vi "AR Drone - Simple Video + Simple nav.vi"() -> ()   [LabVIEW 2014]
doc: "Very simple example showing how to use the base VIs to control the AR Drone and receive and display video data."
uses:
  Others (.ctl)/Control cluster.ctl
  <vilib>/LVH/AR Drone Toolkit/Decode NavData/Typedefs/NavData Demo.ctl
  Global.vi
  <vilib>/LVH/AR Drone Toolkit/AR Drone.lvlib
panel:
  out "error":bool
  out "Take off/Land":bool
  in  "video refresh (ms)":u32=40
  out "Refesh Rate Video Loop (ms) 2":u32
  out "Refesh Rate (ms)":u32=5
  out "Hover":bool
  in  "Tab Control":enum32{"Page 1", "Page 2"}(tab)
  out "B&W":T1(plugin-control)
  out "Raw":picture
  in  "Manual":bool=TRUE
  in  "Setup Parameters":T2={"Drone IP address"="192.168.1.1", "Home IP address"="192.168.1.2", "Flight Mode"=enum."INDOOR MODE", "Mounted Hull"=enum."INDOOR HULL", "Video Camera"=0, "Max Altitude (m)"=3.0, "Max Pitch and Roll Angle (deg)"=8.0, "Max Vertical Speed (m/s)"=0.7, "Max Yaw Speed (deg/s)"=100.0} {"Video Camera" items=["Bottom Camera"=1, "Front Camera"=0, "Front in Bottom"=3, "Bottom in Front"=2]}
  in  "stop":bool
  in  "milliseconds to wait":u32=10
  out "ctr+nav":errorcluster
  out "ctr+nav":i32=2242
  out "Battery Remaining 2":dbl(slide)=55.0 scale=0.0..100.0
  out "NavData Out 2":T3={"control state"=enum."TRANS_LANDING", "battery percentage"=55, "pitch (deg)"=-0.02, "roll (deg)"=0.087, "yaw (deg)"=91.646, "altitude (cm)"=0, "vx (cm/s)?"=0.0, "vy (cm/s)?"=0.0, "vz (cm/s)?"=0.0, "detection cam type"=3}
  out "Control Cluster":T4={"Roll"=0.0, "Pitch"=-0.10223389, "Vertical Speed"=0.0, "Yaw Speed"=0.0} {"Yaw Speed" scale=-1.0..1.0; "Vertical Speed" scale=-1.0..1.0; "Pitch" scale=-1.0..1.0; "Roll" scale=-1.0..1.0}
  in  "Emergency Landing":bool
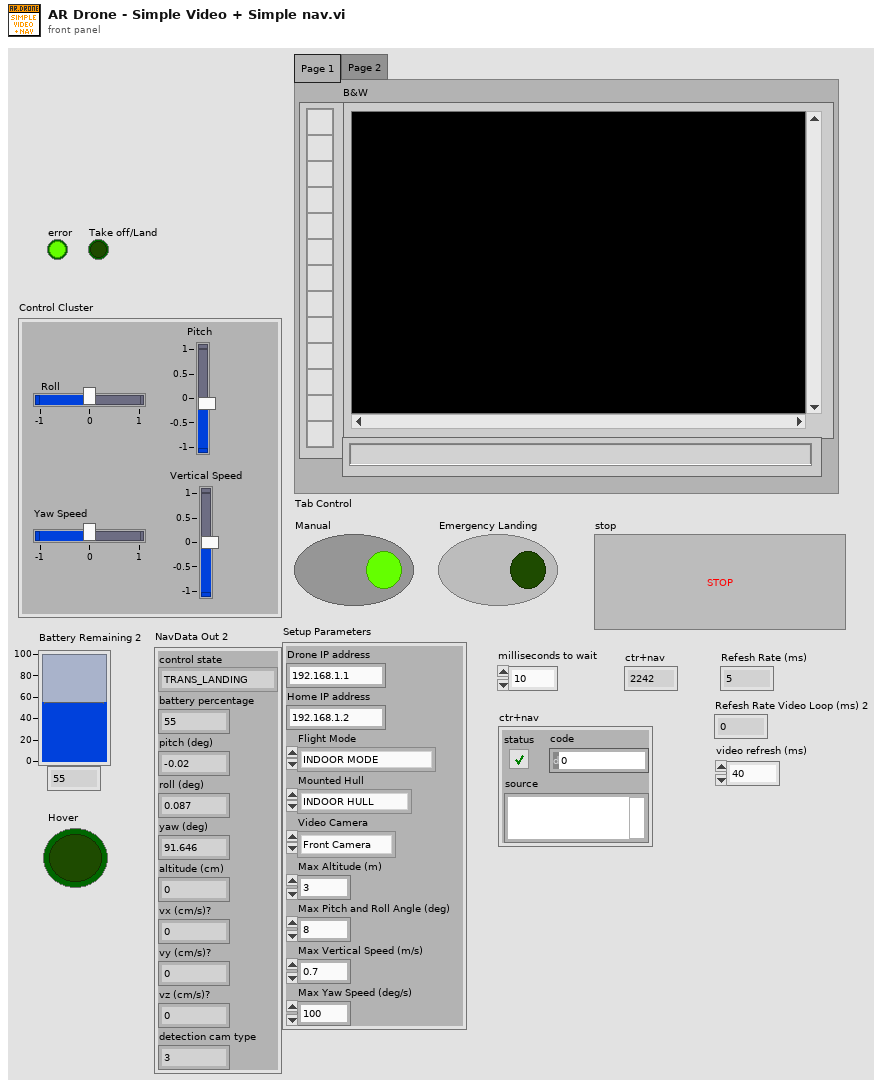
[diagram p1: front panel]
types:
  T1 = typedef "IMAQ Image.ctl" = refnum<image>
  T2 = cluster{"Drone IP address":string, "Home IP address":string, "Flight Mode":enum8{"OUTDOOR MODE", "INDOOR MODE"}, "Mounted Hull":enum8{"OUTDOOR HULL", "INDOOR HULL"}, "Video Camera":u8, "Max Altitude (m)":sgl, "Max Pitch and Roll Angle (deg)":sgl, "Max Vertical Speed (m/s)":sgl, "Max Yaw Speed (deg/s)":sgl}
  T3 = typedef "AR Drone.lvlib/NavData Demo.ctl" = cluster{"control state":enum32{"DEFAULT", "INIT", "LANDING", "FLYING", "HOVERING", "TEST", "TRANS_TAKEOFF", "TRANS_GOTOFIX", "TRANS_LANDING"}, "battery percentage":u32, "pitch (deg)":sgl, "roll (deg)":sgl, "yaw (deg)":sgl, "altitude (cm)":u32, "vx (cm/s)?":sgl, "vy (cm/s)?":sgl, "vz (cm/s)?":sgl, "detection cam type":u32}
  T4 = typedef "Control cluster.ctl" = cluster{"Roll":sgl, "Pitch":sgl, "Vertical Speed":sgl, "Yaw Speed":sgl}
  T5 = typedef "AR Drone.lvlib/AR Drone Resource.ctl" = cluster{"UDP Control Connection":refnum<k16>, "UDP NavData Connection":refnum<k16>, "UDP Video Connection (Drone 1.0)":refnum<k16>, "TCP Video Connection (Drone 2.0)":refnum<k5>, "TCP Control Port Connection":refnum<k5>, "Drone IP address":string, "Drone Command Port":u16, "Drone NavData Port":u16, "Drone Vid Stream Port":u16, "Drone TCP Control Port":u16, "Home IP address":string, "Home Command Port":u16, "Home NavData Port":u16, "Home Vid Stream Port":u16, "Drone Version":i32, "Drone Index":i32, "Command Sequence":i32}
  T6 = cluster{"button 1":bool, "button 2":bool, "button 3":bool, "button 4":bool}
  T7 = cluster{"Roll":dbl, "Pitch":dbl, "Vertical Speed":dbl, "Yaw Speed":dbl}
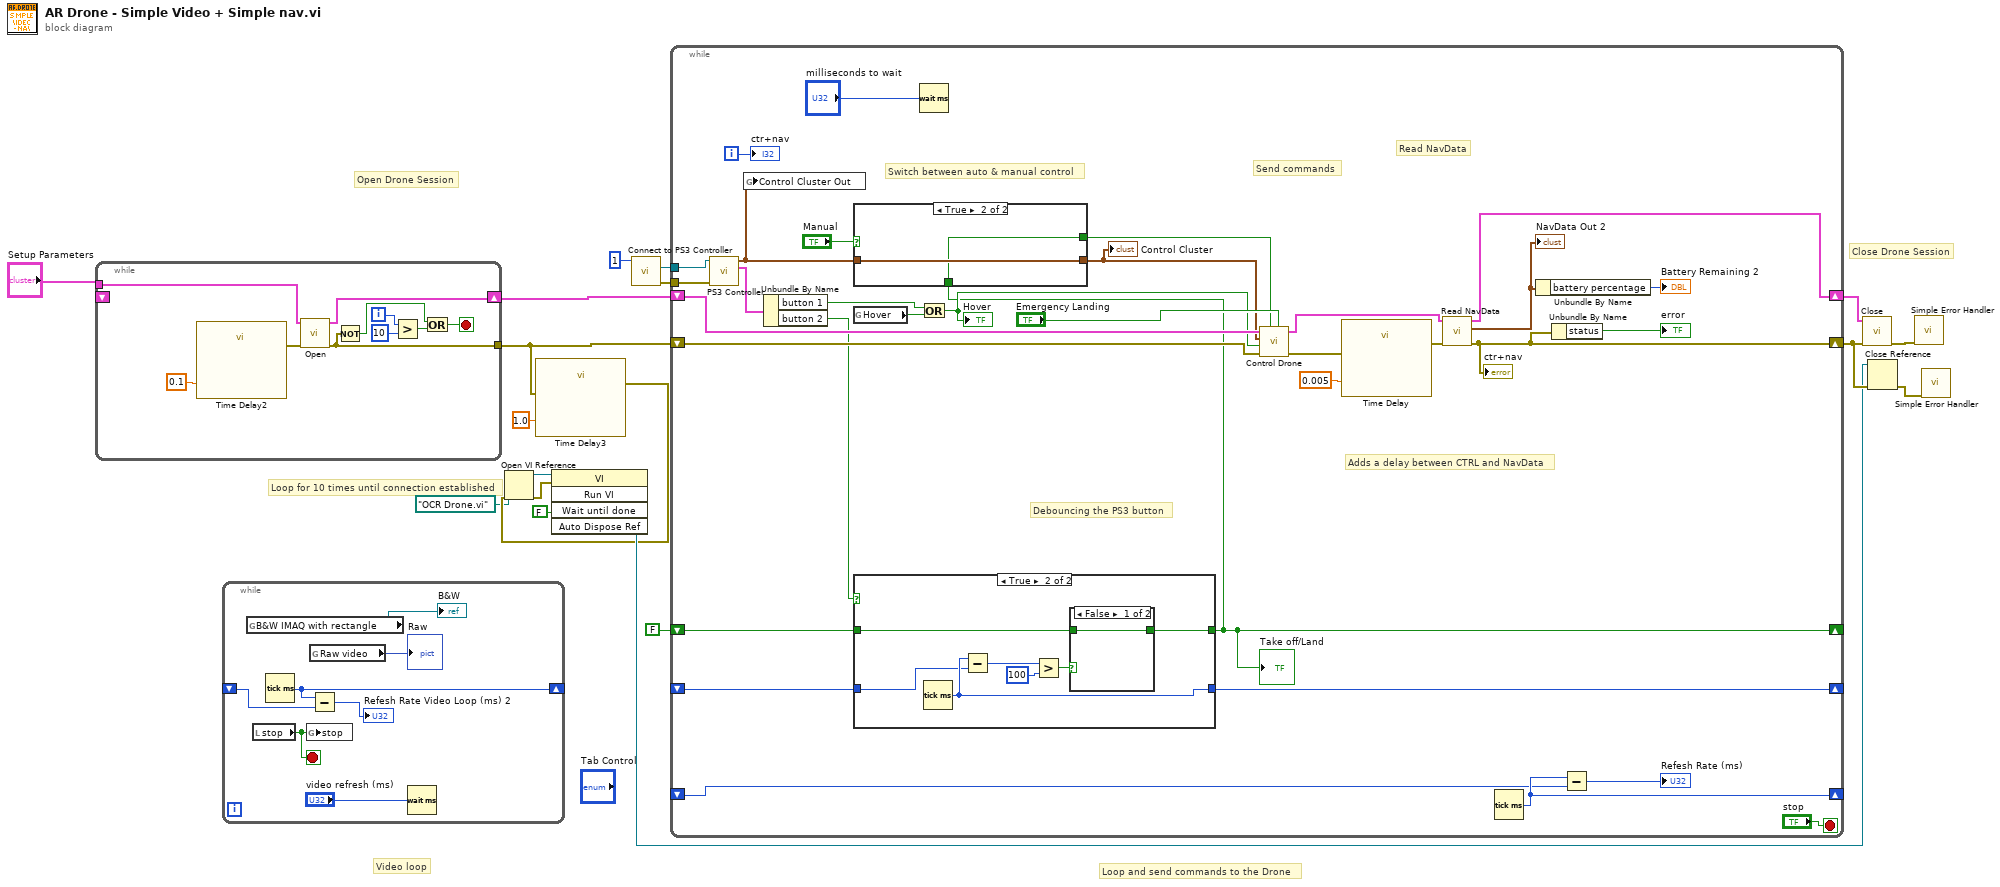
[diagram p0: block diagram]
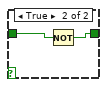
[diagram p3: hidden frame]
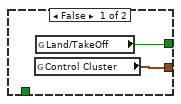
[diagram p4: hidden frame]
diagram:
  # "Loop for 10 times until connection established"
  # "Video loop"
  # "Close Drone Session"
  # "Loop and send commands to the Drone"
  # "Open Drone Session"
  n1 = while {
    tunnel: [w19] -> w10
    tunnel: "Setup Parameters" -> [w27]
    shift-right: [w28] -> w13
    shift-left: _ -> [_]
    i -> [w23]
    stop <- w25 stop-if-true
    n2 = call "Time Delay2"("Delay Time (s)"=0.1) -> ("error out"=w20:errorcluster)  [unwired: 10 in]
    n3 = call <vilib>:"Open.vi"("error in (no error)"=w20, "Setup Parameters"=w27) -> ("error out"=w19:errorcluster, "AR Drone Resource"=w28:T5)  [unwired: 8 in]
    n4 = Not(x=w19) -> (.not. x?=w21:bool)
    n5 = Greater?(x=w23, y=10) -> (0:w24:bool)
    n6 = Or(x=w21, y=w24) -> (x .or. y?=w25:bool)
  }
  n7 = while {
    shift-right: [w33] -> _
    shift-left: _ -> [w32]
    stop <- w29 stop-if-true
    n8 = global read "Global.vi" "B&W IMAQ with rectangle"() -> (→"B&W":T1)
    n9 = local read "stop"() -> (w29:bool)
    n10 = Tick Count (ms)() -> (millisecond timer value=w33:u32)
    n11 = global write "Global.vi" "stop"(w29) -> ()
    n12 = global read "Global.vi" "Raw video"() -> (→"Raw":picture)
    n13 = Subtract(x=w33, y=w32) -> (x-y=→"Refesh Rate Video Loop (ms) 2":u32)
    n14 = Wait (ms)(milliseconds to wait="video refresh (ms)") -> ()  [unwired: 1 out]
  }
  n15 = call "Time Delay3"("error in (no error)"=w10, "Delay Time (s)"=1.0) -> ("error out"=w3:errorcluster)  [unwired: 9 in]
  n16 = Open VI Reference(vi path=path "OCR Drone.vi", error in (no error)=w3) -> (vi reference=w6:refnum<vi>, error out=w4:errorcluster)  [unwired: 4 in]
  n17 = invoke class="VI" method="Run VI"(reference=w6, error in=w4, "Wait until done"=FALSE) -> (reference out=w7:refnum<vi>)  [unwired: 2 in, 4 out]
  n18 = call "Connect to PS3 Controller.vi"("device ID"=1) -> ("error out"=w14:errorcluster, "device ID 2"=w16:refnum<k1>)  [unwired: 7 in, 1 out]
  n19 = while {
    shift-right: [w67] -> w18
    shift-left: w13 -> [w64]
    shift-right: [w60] -> w8
    shift-left: w10 -> [w65]
    tunnel: w16 -> [w62]
    tunnel: w14 -> [w61]
    shift-right: [w51] -> _
    shift-left: _ -> [w50]
    shift-right: [w36] -> _
    shift-left: FALSE -> [w48]
    shift-right: [w47] -> _
    shift-left: _ -> [w46]
    i -> [w63]
    stop <- "stop" stop-if-true
    # "Read NavData"
    # "Send commands"
    # "Switch between auto & manual control"
    # "Debouncing the PS3 button"
    # "Adds a delay between CTRL and NavData"
    n20 = call "PS3 Controller.vi"("error in (no error)"=w61, "device ID"=w62) -> ("Buttons control"=w59:T6, "Control cluster"=w44:T7)  [unwired: 6 in, 2 out]
    n21 = global write "Global.vi" "Control Cluster Out"(w44) -> ()
    n22 = Unbundle By Name(w59) -> ("button 1"=w54:bool, "button 2"=w49:bool)
    n23 = global read "Global.vi" "Hover"() -> (w53:bool)
    n24 = case shown="True" w49 {
      tunnel: [w70 w71] -> w36
      tunnel: w48 -> [w70 w72]
      tunnel: [w69 w77] -> w47
      tunnel: w46 -> [w69 w76]
      frame False {
      }
      frame True {
        n25 = Tick Count (ms)() -> (millisecond timer value=w77:u32)
        n26 = Subtract(x=w77, y=w76) -> (x-y=w75:u32)
        n27 = Greater?(x=w75, y=u32 100) -> (0:w73:bool)
        n28 = case shown="False" w73 {
          tunnel: w72 -> [w78 w80]
          tunnel: [w78 w79] -> w71
          frame False {
          }
          frame True {
            n29 = Not(x=w80) -> (.not. x?=w79:bool)
          }
        }
      }
    }
    "Take off/Land" <- w36
    n30 = case shown="True" "Manual" {
      tunnel: w44 -> [_ w84]
      tunnel: [w82 w84] -> w45
      tunnel: [w81 w83] -> w37
      tunnel: w36 -> [_ w83]
      frame False {
        n31 = global read "Global.vi" "Control Cluster"() -> (w82:T4)
        n32 = global read "Global.vi" "Land/TakeOff"() -> (w81:bool)
      }
      frame True {
      }
    }
    "Control Cluster" <- w45
    n33 = Wait (ms)(milliseconds to wait="milliseconds to wait") -> ()  [unwired: 1 out]
    n34 = Or(x=w54, y=w53) -> (x .or. y?=w52:bool)
    "Hover" <- w52
    n35 = call <vilib>:"Control Drone.vi"("Emergency Landing"="Emergency Landing", "Takeoff/Land"=w37, "error in (no error)"=w65, "Hover"=w52, "Control Cluster"=w45, "AR Drone Resource"=w64) -> ("error out"=w41:errorcluster, "AR Drone Resource Out"=w58:T5)  [unwired: 4 in]
    n36 = call "Time Delay"("error in (no error)"=w41, "Delay Time (s)"=0.005) -> ("error out"=w40:errorcluster)  [unwired: 9 in]
    n37 = call <vilib>:"Read NavData.vi"("error in (no error)"=w40, "AR Drone Resource"=w58) -> ("error out"=w60:errorcluster, "NavData Out"=w56:T3, "AR Drone Resource Out"=w67:T5)  [unwired: 7 in]
    "ctr+nav" <- w60
    "NavData Out 2" <- w56
    n38 = Tick Count (ms)() -> (millisecond timer value=w51:u32)
    n39 = Unbundle By Name(w56) -> ("battery percentage"=→"Battery Remaining 2":u32)
    n40 = Unbundle By Name(w60) -> ("status"=→"error":bool)
    n41 = Subtract(x=w51, y=w50) -> (x-y=→"Refesh Rate (ms)":u32)
    "ctr+nav" <- w63
  }
  n42 = call <vilib>:"Close.vi"("error in (no error)"=w8, "AR Drone Resource"=w18) -> ("error out"=w17:errorcluster)  [unwired: 9 in]
  n43 = Close Reference(reference=w7, error in (no error)=w8) -> (error out=w1:errorcluster)
  n44 = call <vilib>:"Simple Error Handler.vi"("error in (no error)"=w17) -> ()  [unwired: 4 in, 5 out]
  n45 = call <vilib>:"Simple Error Handler.vi"("error in (no error)"=w1) -> ()  [unwired: 4 in, 5 out]
